vi "135-lvlib-p_path.vi"(8 "error in (no error)":errorcluster) -> (0 "error out":errorcluster)   [LabVIEW 2020]
uses:
  classes/Assert/Assert Equal Value_Variant.vi
  classes/Test/Test.lvclass
  classes/Assert/Assert.lvclass
  Caraya.lvlib
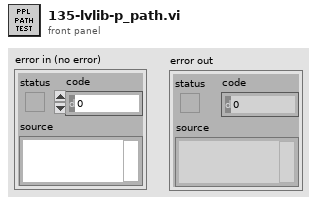
[diagram p1: front panel]
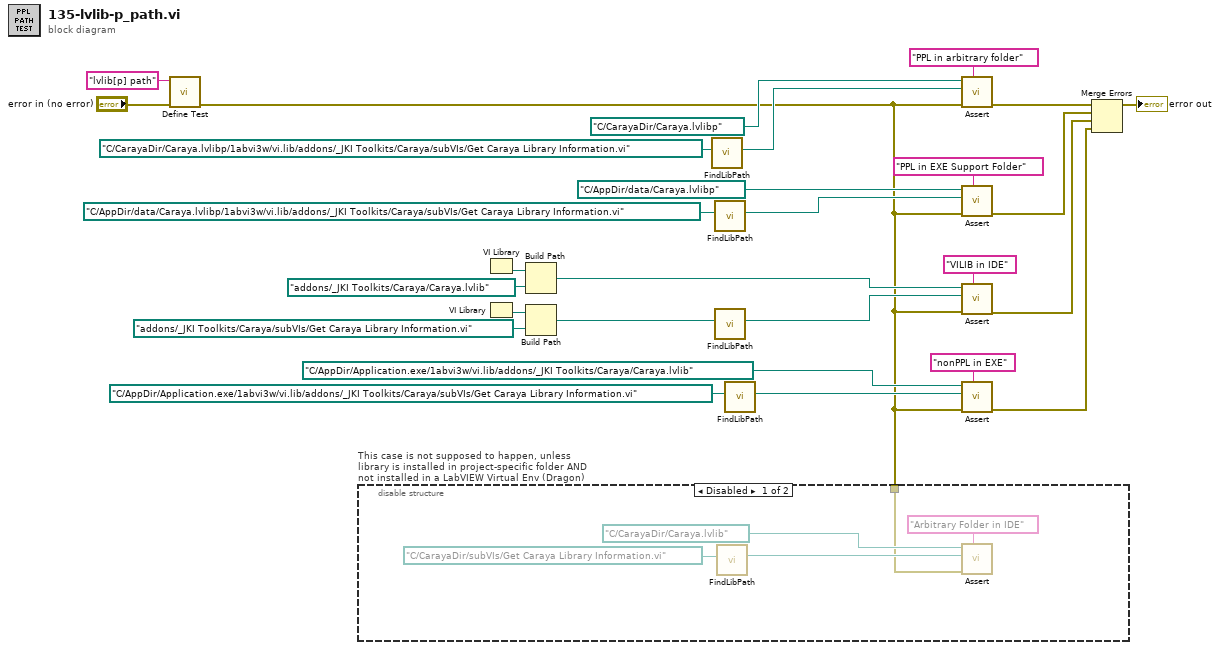
[diagram p0: block diagram]
diagram:
  n1 = call "Define Test.vi"("error in (no error)"="error in (no error)", "Label (VI Title)"="lvlib[p] path") -> ("error out"=w1:errorcluster)  [unwired: 8 in, 1 out]
  n2 = disable-structure "This case is not supposed to happen, unless library is installed in project-specific folder AND not installed in a LabVIEW Virtual Env (Dragon)" shown="Disabled" {
    disable-tunnel: w1 -> [w29 _]
    frame Disabled {
      n3 = call "FindLibPath.vi"("Caraya Library Member Path"=path "C:/CarayaDir/subVIs/Get Caraya Library Information.vi") -> ("Caraya Library Path"=w30:path)  [unwired: 10 in]
      n4 = call-poly "Assert.vi"("Label"="Arbitrary Folder in IDE", "error in (no error)"=w29, "Y"=w30, "X"=path "C:/CarayaDir/Caraya.lvlib") -> ()  [unwired: 6 in, 2 out]
    }
    frame Enabled {
    }
  }
  n5 = VI Library() -> (path=w20:path)
  n6 = VI Library() -> (path=w19:path)
  n7 = Build Path(base path=w20, name or relative path=path "addons/_JKI Toolkits/Caraya/Caraya.lvlib") -> (appended path=w6:path)
  n8 = Build Path(base path=w19, name or relative path=path "addons/_JKI Toolkits/Caraya/subVIs/Get Caraya Library Information.vi") -> (appended path=w17:path)
  n9 = call "FindLibPath.vi"("Caraya Library Member Path"=path "C:/CarayaDir/Caraya.lvlibp/1abvi3w/vi.lib/addons/_JKI Toolkits/Caraya/subVIs/Get Caraya Library Information.vi") -> ("Caraya Library Path"=w23:path)  [unwired: 10 in]
  n10 = call "FindLibPath.vi"("Caraya Library Member Path"=path "C:/AppDir/data/Caraya.lvlibp/1abvi3w/vi.lib/addons/_JKI Toolkits/Caraya/subVIs/Get Caraya Library Information.vi") -> ("Caraya Library Path"=w7:path)  [unwired: 10 in]
  n11 = call "FindLibPath.vi"("Caraya Library Member Path"=w17) -> ("Caraya Library Path"=w5:path)  [unwired: 10 in]
  n12 = call "FindLibPath.vi"("Caraya Library Member Path"=path "C:/AppDir/Application.exe/1abvi3w/vi.lib/addons/_JKI Toolkits/Caraya/subVIs/Get Caraya Library Information.vi") -> ("Caraya Library Path"=w3:path)  [unwired: 10 in]
  n13 = call-poly "Assert.vi"("Label"="PPL in arbitrary folder", "error in (no error)"=w1, "Y"=w23, "X"=path "C:/CarayaDir/Caraya.lvlibp") -> ("error out"=w13:errorcluster)  [unwired: 6 in, 1 out]
  n14 = call-poly "Assert.vi"("Label"="PPL in EXE Support Folder", "error in (no error)"=w1, "Y"=w7, "X"=path "C:/AppDir/data/Caraya.lvlibp") -> ("error out"=w11:errorcluster)  [unwired: 6 in, 1 out]
  n15 = call-poly "Assert.vi"("Label"="VILIB in IDE", "error in (no error)"=w1, "Y"=w5, "X"=w6) -> ("error out"=w10:errorcluster)  [unwired: 6 in, 1 out]
  n16 = call-poly "Assert.vi"("Label"="nonPPL in EXE", "error in (no error)"=w1, "Y"=w3, "X"=path "C:/AppDir/Application.exe/1abvi3w/vi.lib/addons/_JKI Toolkits/Caraya/Caraya.lvlib") -> ("error out"=w9:errorcluster)  [unwired: 6 in, 1 out]
  n17 = Merge Errors(w13, w11, w10, w9) -> (→"error out":errorcluster)
